vi "Identify Oxford.vi"(8 "Error In":errorcluster, 11 "VISA resource name":refnum<visa-resource-name>) -> (0 "Error Out":errorcluster, 1 "read buffer":string, 2 "It's from Oxford!":bool, 3 "VISA resource name out":refnum<visa-resource-name>, 5 "Instrument":T1)   [LabVIEW 2016]
uses:
  Device/Device type.ctl
  Oxford crappy logic options.ctl
  GPIB/VISA  Send Receive.vi
panel:
  out "dump buffer serial":string
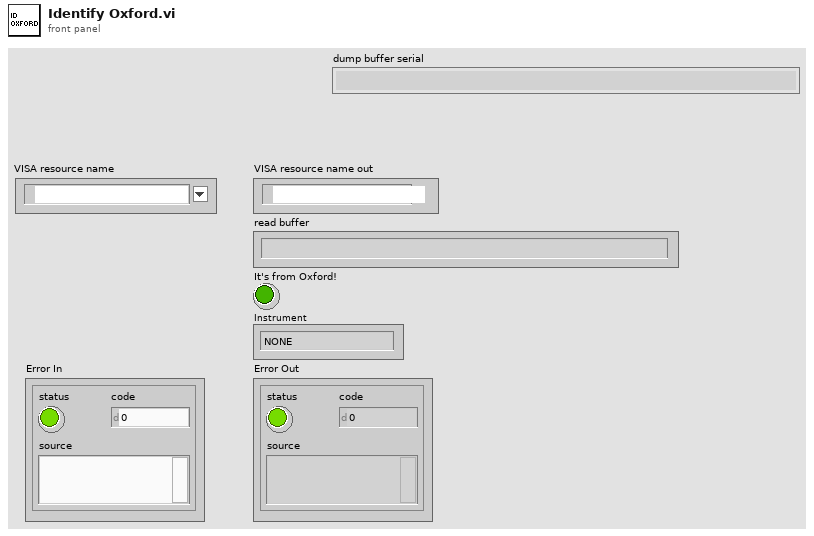
[diagram p1: front panel]
types:
  T1 = typedef "Device type.ctl" = enum16{"NONE", "Neocera 21", "LakeShore 335", "LakeShore 336", "LakeShore 340", "LkShr 340 chA&B", "LakeShore 370", "SRS 850", "SRS 830", "LR 700", "EG&G 5302", "EG&G 7260", "EG&G 7280", "AH 2500", "Keithley meter", "Keithley electrometer", "Keithley 182", "HP 5385", "HP 53181", "HP 53132", "ITC503", "IPS120", "Oxford Mercury IPS", "Oxford PS", "Test", "DC Facility Magnet", "Cryomagnetics PS", "Keithley 2400", "Keithley current source", "Cryo-Con 22C", "HP87NN", "HP4395A", "Agilent 34410A"}
  T2 = typedef "Oxford crappy logic options.ctl" = enum16{"Unknown", "Serial PS", "ITC-503"}
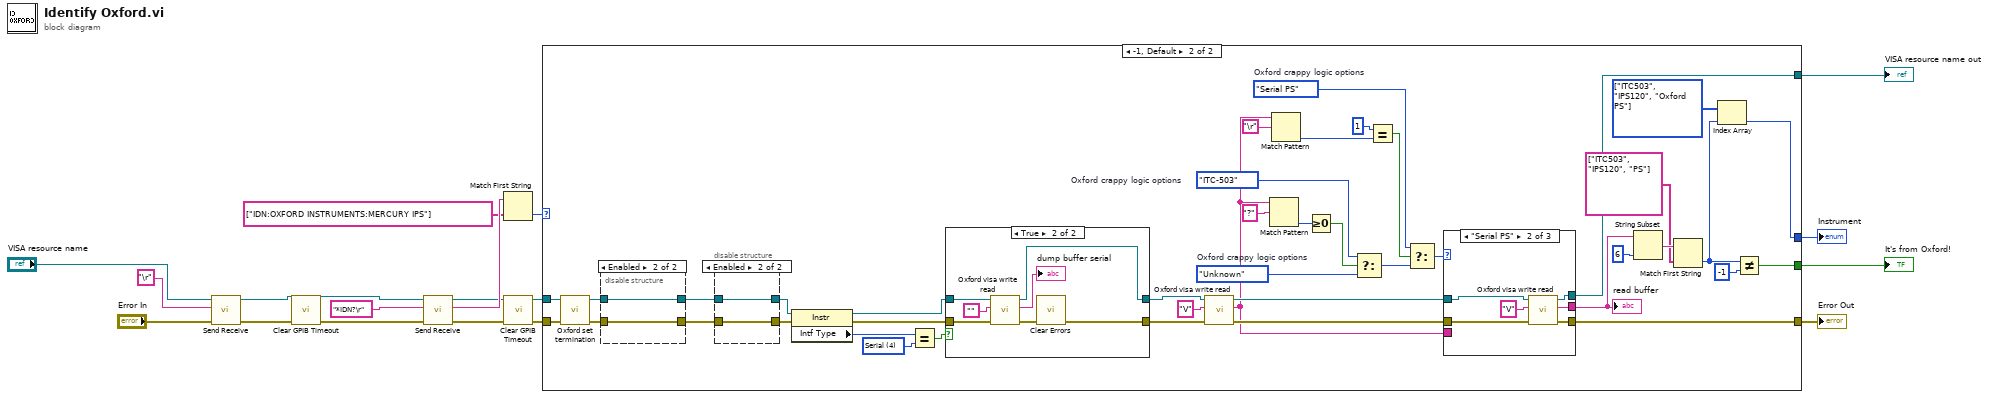
[diagram p0: block diagram]
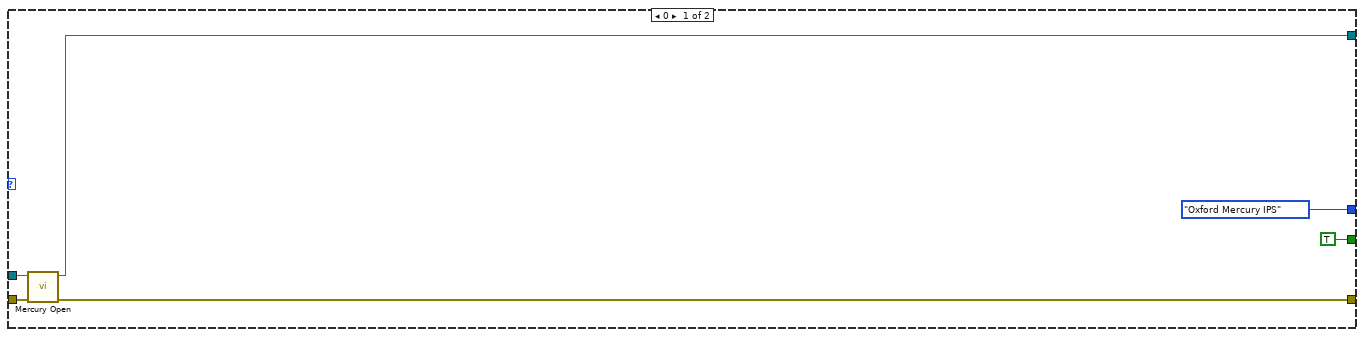
[diagram p2: hidden frame]
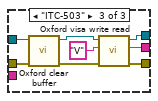
[diagram p4: hidden frame]
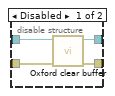
[diagram p6: hidden frame]
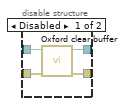
[diagram p7: hidden frame]
diagram:
  n1 = call-poly "Send Receive.vi"("error in (no error)"="Error In", "data string in"="\r" ("data string"), "VISA Resource Name"="VISA resource name") -> ("error out"=w4:errorcluster, "VISA Resource Name Out"=w7:refnum<visa-resource-name>)  [unwired: 6 in, 1 out]
  n2 = call "Clear GPIB Timeout.vi"("error in (no error)"=w4) -> ("error out"=w5:errorcluster)  [unwired: 1 in, 9 out]
  n3 = call-poly "Send Receive.vi"("error in (no error)"=w5, "data string in"="*IDN?\r" ("data string"), "VISA Resource Name"=w7) -> ("error out"=w13:errorcluster, "data string out"=w11:string, "VISA Resource Name Out"=w10:refnum<visa-resource-name>)  [unwired: 6 in]
  n4 = Match First String(2:string[] ["IDN:OXFORD INSTRUMENTS:MERCURY IPS"] ("string array"), 3:w11) -> (0:w8:i32)  [unwired: 1 out]
  n5 = call "Clear GPIB Timeout.vi"("error in (no error)"=w13) -> ("error out"=w14:errorcluster)  [unwired: 1 in, 9 out]
  n6 = case shown="-1, Default" w8 {
    tunnel: [w20 w36] -> w17
    tunnel: [TRUE w58] -> w16
    tunnel: [Device_type."Oxford Mercury IPS" ("Instrument") w55] -> w15
    tunnel: w14 -> [w19 w43]
    tunnel: w10 -> [w21 w42]
    tunnel: [w18 w37] -> w1
    frame 0 {
      n7 = call "Mercury Open.vi"("Error In"=w19, "VISA resource name"=w21) -> ("Error Out"=w18:errorcluster, "VISA resource name out"=w20:refnum<visa-resource-name>)  [unwired: 8 in]
    }
    frame -1, Default {
      w27 = Oxford_crappy_logic_options."ITC-503"  # Oxford crappy logic options
      w29 = Oxford_crappy_logic_options."Serial PS"  # Oxford crappy logic options
      w28 = Oxford_crappy_logic_options."Unknown"  # Oxford crappy logic options
      w45 = u16 4 items=["GPIB"=1, "VXI"=2, "GPIB-VXI"=3, "Serial"=4, "PXI"=5, "TCPIP"=6, "USB"=7, "FireWire"=9] ("Interface Information:Interface Type")
      w57 = T1[] [enum."ITC503", enum."IPS120", enum."Oxford PS"] items=["NONE", "Neocera 21", "LakeShore 335", "LakeShore 336", "LakeShore 340", "LkShr 340 chA&B", "LakeShore 370", "SRS 850", "SRS 830", "LR 700", "EG&G 5302", "EG&G 7260", "EG&G 7280", "AH 2500", "Keithley meter", "Keithley electrometer", "Keithley 182", "HP 5385", "HP 53181", "HP 53132", "ITC503", "IPS120", "Oxford Mercury IPS", "Oxford PS", "Test", "DC Facility Magnet", "Cryomagnetics PS", "Keithley 2400", "Keithley current source", "Cryo-Con 22C", "HP87NN", "HP4395A", "Agilent 34410A"] ("Array")
      n8 = call "Oxford set termination.vi"("error in (no error)"=w43, "VISA resource name"=w42) -> ("error out"=w54:errorcluster, "VISA resource name out"=w53:refnum<visa-resource-name>)  [unwired: 8 in]
      n9 = disable-structure shown="Enabled" {
        disable-tunnel: w54 -> [w95 w96]
        disable-tunnel: [w94 w96] -> w63
        disable-tunnel: w53 -> [w92 w97]
        disable-tunnel: [w93 w97] -> w62
        frame Disabled {
          n10 = call "Oxford clear buffer.vi"("error in (no error)"=w95, "VISA resource name"=w92) -> ("error out"=w94:errorcluster, "VISA resource name out"=w93:refnum<visa-resource-name>)  [unwired: 6 in, 2 out]
        }
        frame Enabled {
        }
      }
      n11 = disable-structure shown="Enabled" {
        disable-tunnel: w62 -> [w101 w102]
        disable-tunnel: [w100 w102] -> w50
        disable-tunnel: w63 -> [w99 w103]
        disable-tunnel: [w98 w103] -> w48
        frame Disabled {
          n12 = call "Oxford clear buffer.vi"("error in (no error)"=w99, "VISA resource name"=w101) -> ("error out"=w98:errorcluster, "VISA resource name out"=w100:refnum<visa-resource-name>)  [unwired: 6 in, 2 out]
        }
        frame Enabled {
        }
      }
      n13 = property class="Instr"(reference=w50, error in=w48) -> (reference out=w49:refnum<visa-resource-name>, error out=w47:errorcluster, "Intf Type"=w46:u16)
      n14 = Equal?(x=w46, y=w45) -> (x = y?=w44:bool)
      n15 = case shown="True" w44 {
        tunnel: [w84 w90] -> w52
        tunnel: [w83 w86] -> w51
        tunnel: w49 -> [w84 w88]
        tunnel: w47 -> [w83 w87]
        frame False {
        }
        frame True {
          n16 = call "Oxford visa write read.vi"("error in (no error)"=w87, "write buffer"="", "VISA resource name"=w88) -> ("error out"=w89:errorcluster, "read buffer"=→"dump buffer serial":string, "VISA resource name out"=w90:refnum<visa-resource-name>)  [unwired: 6 in]
          n17 = call <vilib>:"Clear Errors.vi"("error in (no error)"=w89) -> ("error out"=w86:errorcluster)  [unwired: 5 in, 1 out]
        }
      }
      n18 = call "Oxford visa write read.vi"("error in (no error)"=w51, "write buffer"="V", "VISA resource name"=w52) -> ("error out"=w38:errorcluster, "read buffer"=w33:string, "VISA resource name out"=w39:refnum<visa-resource-name>)  [unwired: 6 in]
      n19 = Match Pattern(string=w33, regular expression="?") -> (offset past match=w40:i32)  [unwired: 1 in, 3 out]
      n20 = Match Pattern(string=w33, regular expression="\r") -> (offset past match=w32:i32)  [unwired: 1 in, 3 out]
      n21 = Greater Or Equal To 0?(x=w40) -> (x >= 0?=w26:bool)
      n22 = Select(t=w27, s=w26, f=w28) -> (s? t:f=w25:T2)
      n23 = Equal?(x=1, y=w32) -> (x = y?=w30:bool)
      n24 = Select(t=w29, s=w30, f=w25) -> (s? t:f=w24:T2)
      n25 = case shown="\"Serial PS\"" w24 {
        tunnel: w39 -> [w68 w69 w82]
        tunnel: w38 -> [w67 w73 w81]
        tunnel: [w67 w72 w78] -> w37
        tunnel: [w68 w71 w76] -> w36
        tunnel: [w66 w70 w75] -> w35
        tunnel: w33 -> [w66 _ _]
        frame "Unknown", Default {
        }
        frame "Serial PS" {
          n26 = call "Oxford visa write read.vi"("error in (no error)"=w73, "write buffer"="V", "VISA resource name"=w69) -> ("error out"=w72:errorcluster, "read buffer"=w70:string, "VISA resource name out"=w71:refnum<visa-resource-name>)  [unwired: 6 in]
        }
        frame "ITC-503" {
          n27 = call "Oxford clear buffer.vi"("error in (no error)"=w81, "VISA resource name"=w82) -> ("error out"=w79:errorcluster, "VISA resource name out"=w77:refnum<visa-resource-name>)  [unwired: 6 in, 2 out]
          n28 = call "Oxford visa write read.vi"("error in (no error)"=w79, "write buffer"="V", "VISA resource name"=w77) -> ("error out"=w78:errorcluster, "read buffer"=w75:string, "VISA resource name out"=w76:refnum<visa-resource-name>)  [unwired: 6 in]
        }
      }
      "read buffer" <- w35
      n29 = String Subset(string=w35, length (rest)=6 ("length (rest)")) -> (substring=w61:string)  [unwired: 1 in]
      n30 = Match First String(2:string[] ["ITC503", "IPS120", "PS"], 3:w61) -> (0:w56:i32)  [unwired: 1 out]
      n31 = Index Array(array=w57, index=w56) -> (element=w55:T1)
      n32 = Not Equal?(x=w56, y=-1) -> (x != y?=w58:bool)
    }
  }
  "VISA resource name out" <- w17
  "It's from Oxford!" <- w16
  "Instrument" <- w15
  "Error Out" <- w1
